vi "GetDigitalOutputStatus.vi"(0 "VISA resource name":refnum<visa-resource-name>, 5 "control module number":T1=1 items=["control module 1"=1, "control module 2"=2, "control module 3"=3, "control module 4"=4], 9 "Extended?":bool, 11 "error in":errorcluster) -> (4 "VISA resource name out":refnum<visa-resource-name>, 6 "Digital Output Status string":string, 8 "Digital Output Status":i32, 10 "Digital Output Status binary":string, 15 "error out":errorcluster)   [LabVIEW 2023, in "Thermotron 8800.lvlib"]
doc: "DIGO\nCommand name: Send digital output (DO) status\nCommand type: System status\nDescription: This command returns either a 24-bit integer value that indicates which of digital\noutputs 1 through 24 are active, or a 16-bit integer value that indicates which of\ndigital outputs 25 through 40 are active. You must use the letter “e” to get the status\nof digital outputs 25 through 40.\nStandard digital outputs:\nDO 6 DO 5 DO 4 DO 3 DO 2 DO 1\nbit 5 bit 4 bit 3 bit 2 bit 1 bit 0\nDO 12 DO 11 DO 10 DO 9 DO 8 DO 7\nbit 11 bit 10 bit 9 bit 8 bit 7 bit 6\nDO 18 DO 17 DO 16 DO 15 DO 14 DO 13\nbit 17 bit 16 bit 15 bit 14 bit 13 bit 12\nDO 24 DO 23 DO 22 DO 21 DO 20 DO 19\nbit 23 bit 22 bit 21 bit 20 bit 19 bit 18\n\nExtended digital outputs:\nDO 28 DO 27 DO 26 DO 25\nbit 27 bit 26 bit 25 bit 24\nDO 32 DO 31 DO 30 DO 29\nbit 31 bit 30 bit 29 bit 28\nDO 36 DO 35 DO 34 DO 33\nbit 35 bit 34 bit 33 bit 32\nDO 40 DO 39 DO 38 DO 37\nbit 39 bit 38 bit 37 bit 36\nSyntax: DIGOcm,e?\nWhere:\ncm = control module to return (1 through 4)\ne= extended. Use e to return the status of digital outputs 25 through 40.\nQuery example 1: DIGO0?\n8800 response: 2228224 = 001000 100000 000000 000000\nDO 6 DO 5 DO 4 DO 3 DO 2 DO 1\nbit 5: 0 bit 4: 0 bit 3: 0 bit 2: 0 bit 1: 0 bit 0:\nDO 12 DO 11 DO 10 DO 9 DO 8 DO 7\nbit 11: 0 bit 10: 0 bit 9: 0 bit 8: 0 bit 7: 0 bit 6: 0\nDO 18 DO 17 DO 16 DO 15 DO 14 DO 13\nbit 17: 1 bit 16: 0 bit 15: 0 bit 14: 02 bit 13: 0 bit 12: 0\nDO 24 DO 23 DO 22 DO 21 DO 20 DO 19\nbit 23: 0 bit 22: 0 bit 21: 1 bit 20: 0 bit 19: 0 bit 18: 0\n(CM0 digital outputs 18 and 22 are active.)\nQuery example 2: DIGO0,e?\n8800 response: 186 = 0000 0000 1011 1010\nDO 28 DO 27 DO 26 DO 25\nbit 27: 1 bit 26: 0 bit 25: 1 bit 24: 0\nDO 32 DO 31 DO 30 DO 29\nbit 27: 1 bit 30: 0 bit 27: 1 bit 27: 1\nDO 36 DO 35 DO 34 DO 33\nbit 35: 0 bit 34: 0 bit 33: 0 bit 32: 0\nDO 40 DO 39 DO 38 DO 37\nbit 39: 0 bit 38: 0 bit 37: 0 bit 36: 0\n(CM0 digital outputs 26, 28, 29, 30, and 32 are active.)"
uses:
  Thermotron 8800.lvlib
  Private/control module number.ctl
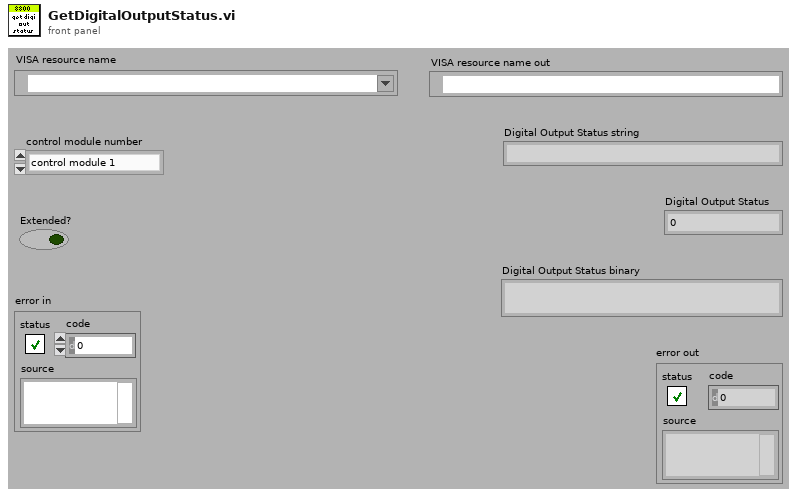
[diagram p1: front panel]
types:
  T1 = typedef "Thermotron 8800.lvlib/control module number.ctl" = u16
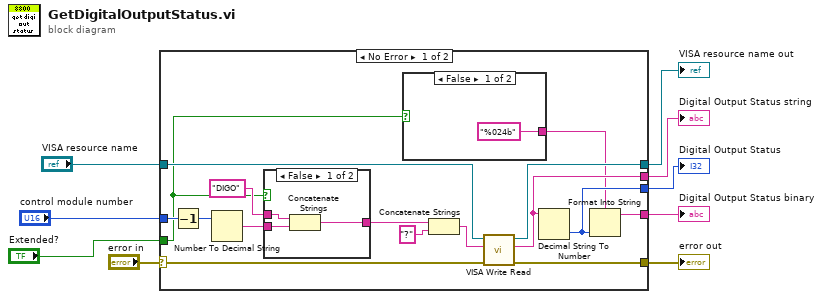
[diagram p0: block diagram]
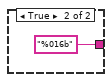
[diagram p2: hidden frame]
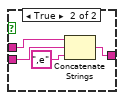
[diagram p3: hidden frame]
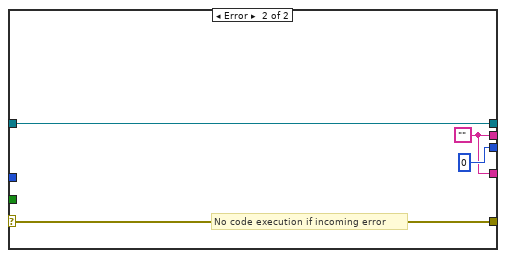
[diagram p4: hidden frame]
diagram:
  n1 = case shown="No Error" "error in" {
    selector: "error in" -> [w24 w38]
    tunnel: [w23 w38] -> w4
    tunnel: "VISA resource name" -> [w22 w36]
    tunnel: [w21 w36] -> w3
    tunnel: [w20 w35] -> w7
    tunnel: [w17 0] -> w8
    tunnel: [w18 w35] -> w9
    tunnel: "Extended?" -> [w11 _]
    tunnel: "control module number" -> [w16 _]
    frame No Error {
      n2 = Decrement(x=w16) -> (x-1=w15:T1)
      n3 = Number To Decimal String(number=w15) -> (decimal integer string=w14:string)  [unwired: 1 in]
      n4 = case shown="False" w11 {
        tunnel: w14 -> [w30 w33]
        tunnel: [w29 w31] -> w13
        tunnel: "DIGO" ("8800 Command") -> [w28 w34]
        frame False {
          n5 = Concatenate Strings(w28, w30) -> (w29:string)
        }
        frame True {
          n6 = Concatenate Strings(w34, w33, ",e" ("8800 Command")) -> (w31:string)
        }
      }
      n7 = case shown="False" w11 {
        tunnel: ["%024b" ("format string") "%016b" ("format string")] -> w10
        frame False {
        }
        frame True {
        }
      }
      n8 = Concatenate Strings(w13, "?" ("8800 Command")) -> (w25:string)
      n9 = call "VISA Write Read.vi"("error in (no error)"=w24, "8800 Command"=w25, "VISA Refnum in"=w22) -> ("error out"=w23:errorcluster, "read buffer"=w20:string, "VISA Refnum out"=w21:refnum<visa-resource-name>)  [unwired: 6 in]
      n10 = Decimal String To Number(string=w20) -> (number=w17:i32)  [unwired: 2 in, 1 out]
      n11 = Format Into String(format string=w10, w17) -> (resulting string=w18:string)  [unwired: 2 in, 1 out]
    }
    frame Error {
      w35 = ""
      # "No code execution if incoming error"
    }
  }
  "VISA resource name out" <- w3
  "error out" <- w4
  "Digital Output Status string" <- w7
  "Digital Output Status" <- w8
  "Digital Output Status binary" <- w9
